vi "FilterArray_Graphic_HP.vi"(4 "Window Size":dbl, 7 "Instantaneous BER":dbl) -> (0 "Slide Bar":dbl, 3 "Graph Instantaneous BER":dbl)   [LabVIEW 2022 SP3]
uses:
  <vilib>/Analysis/baseanly.llb/Mean (DBL).vi
  <vilib>/Analysis/NI_AALBase.lvlib
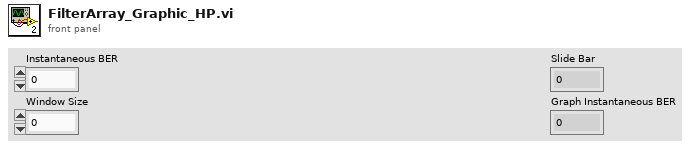
[diagram p1: front panel]
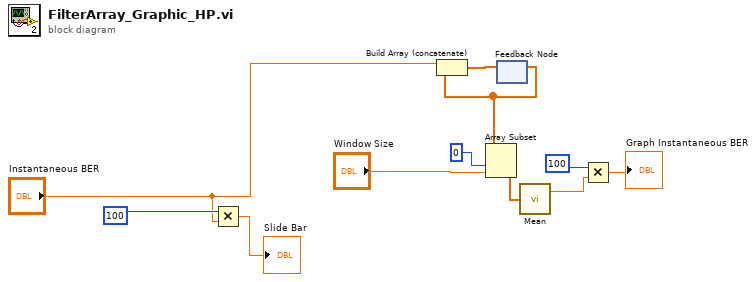
[diagram p0: block diagram]
diagram:
  n1 = Multiply(x=100, y="Instantaneous BER") -> (x*y=→"Slide Bar":dbl)
  n2 = feedback #1() -> (w9:dbl[])  [unwired: 1 in]
  n3 = Build Array (concatenate)("Instantaneous BER", w9) -> (w10:dbl[])
  n4 = Array Subset(array=w9, index=0, length="Window Size") -> (w8:dbl[])
  n5 = feedback-in #1(w10) -> ()
  n6 = call-poly <vilib>:"Mean.vi"("X"=w8) -> ("mean"=w2:dbl)  [unwired: 1 out]
  n7 = Multiply(x=100, y=w2) -> (x*y=→"Graph Instantaneous BER":dbl)
